vi "peak - linear and inverse maps.vi"(8 "4corners":T1={"z (-pi/2)"=-1.0311345636926572+0.5736824521422934i, "z(inf)"=-0.5200164984937075+1.0975277942502903i, "z (pi/2)"=-1.0311345636926572+0.5736824521422934i, "z center"=-0.5136528600391839+0.580046090596817i, "z(0)"=-0.5200164984937075+1.0975277942502903i, "radius"=-1.0311345636926572}, 11 "Z":cdb[](array[numeric])) -> (1 "inverse":cdb[](array[numeric]), 2 "linear":cdb[](array[numeric]))   [LabVIEW 2018]
uses:
  circle corners.ctl
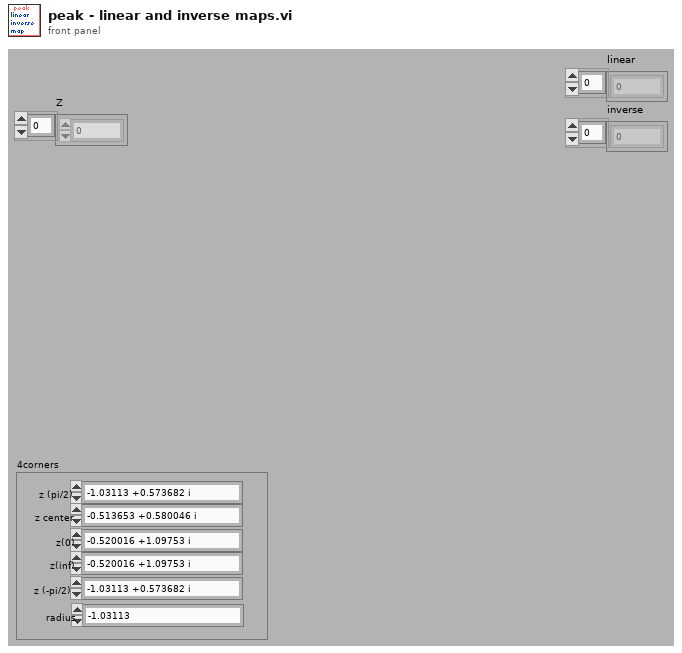
[diagram p1: front panel]
types:
  T1 = typedef "circle corners.ctl" = cluster{"z (-pi/2)":cdb, "z(inf)":cdb, "z (pi/2)":cdb, "z center":cdb, "z(0)":cdb, "radius":dbl}
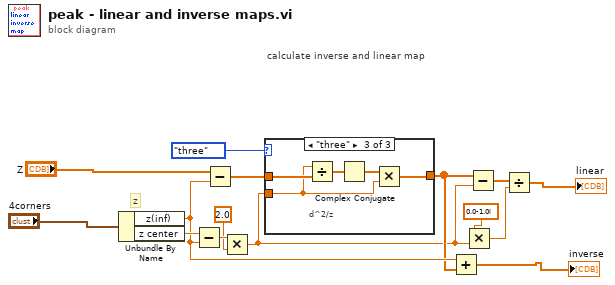
[diagram p0: block diagram]
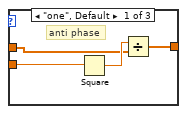
[diagram p2: hidden frame]
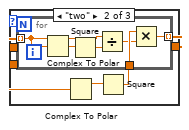
[diagram p3: hidden frame]
diagram:
  # "z"
  # "calculate inverse and linear map"
  n1 = Unbundle By Name("4corners") -> ("z(inf)"=w10:cdb, "z center"=w11:cdb)
  n2 = Subtract(x=w11, y=w10) -> (x-y=w4:cdb)
  n3 = Subtract(x="Z", y=w10) -> (x-y=w5:cdb[])
  n4 = Multiply(x=w4, y=2.0) -> (x*y=w2:cdb)
  n5 = case shown="\"three\"" enum16{"one", "three", "two"}."three" {
    tunnel: w5 -> [w17 w24 w35]
    tunnel: [w16 w21 w31] -> w6
    tunnel: w2 -> [w19 w20 w32]
    frame "one", Default {
      # "anti phase"
      n6 = Square(x=w19) -> (x^2=w18:cdb)
      n7 = Divide(x=w18, y=w17) -> (x/y=w16:cdb[])
    }
    frame "two" {
      n8 = Complex To Polar(r * e^(i*theta)=w20) -> (r=w23:dbl)  [unwired: 1 out]
      n9 = Square(x=w23) -> (x^2=w22:dbl)
      n10 = for {
        tunnel: w24 -> [w30] mode=indexing
        tunnel: w22 -> [w27]
        tunnel: [w25] -> w21 mode=indexing
        n11 = Complex To Polar(r * e^(i*theta)=w30) -> (r=w28:dbl)  [unwired: 1 out]
        n12 = Square(x=w28) -> (x^2=w29:dbl)
        n13 = Divide(x=w30, y=w29) -> (x/y=w26:cdb)
        n14 = Multiply(x=w27, y=w26) -> (x*y=w25:cdb)
      }
    }
    frame "three" {
      # "d^2/z"
      n15 = Divide(x=w32, y=w35) -> (x/y=w34:cdb[])
      n16 = Complex Conjugate(1:w34) -> (0:w33:cdb[])
      n17 = Multiply(x=w33, y=w32) -> (x*y=w31:cdb[])
    }
  }
  n18 = Add(x=w10, y=w6) -> (x+y=→"inverse":cdb[])
  n19 = Multiply(x=cdb 0.0-1.0i ("y"), y=w2) -> (x*y=w8:cdb)
  n20 = Subtract(x=w6, y=w2) -> (x-y=w7:cdb[])
  n21 = Divide(x=w7, y=w8) -> (x/y=→"linear":cdb[])
